vi "Pneumatic Command Initialize.vi"(11 "name (unnamed)":string) -> (2 "RTFIFO Out":u64, 3 "Cluster":T1)   [LabVIEW 2015]
uses:
  <userlib>/836-Library/Pneumatics/Support Code/Pneumatics Notifier.ctl
  <userlib>/836-Library/Pneumatics/Support Code/Pneumatics Command.ctl
  <userlib>/836-Library/Pneumatics/Support Code/Pneumatics Status.ctl
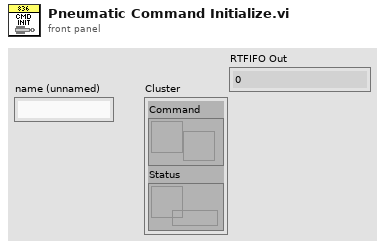
[diagram p1: front panel]
types:
  T1 = typedef "Pneumatics Notifier.ctl" = cluster{"Command":refnum<notifier>, "Status":refnum<queue>}
  T2 = typedef "Pneumatics Command.ctl" = enum16{"Nothing", "Forward", "Reverse", "Toggle"}
  T3 = typedef "Pneumatics Status.ctl" = enum16{"Forward", "Reverse", "Moving"}
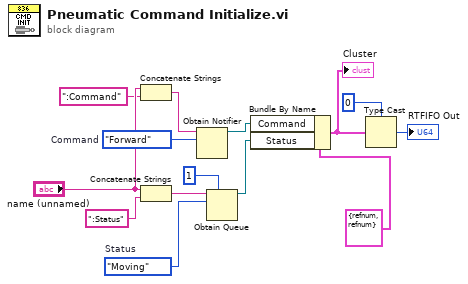
[diagram p0: block diagram]
diagram:
  w12 = Pneumatics_Command."Forward"  # Command
  w11 = Pneumatics_Status."Moving"  # Status
  n1 = Concatenate Strings("name (unnamed)", ":Command" ("string")) -> (w6:string)
  n2 = Concatenate Strings("name (unnamed)", ":Status" ("string")) -> (w9:string)
  n3 = Obtain Notifier(name (unnamed)=w6, notification data type=w12) -> (notifier out=w14:refnum<notifier>)  [unwired: 2 in, 2 out]
  n4 = Obtain Queue(max queue size (-1, unlimited)=1, name (unnamed)=w9, element data type=w11) -> (queue out=w13:refnum<queue>)  [unwired: 2 in, 2 out]
  n5 = Bundle By Name(cluster=T1 {"Command"=refnum, "Status"=refnum}, "Command"=w14, "Status"=w13) -> (w2:T1)
  "Cluster" <- w2
  n6 = Type Cast(type=u64 0, x=w2) -> (*(type *) &x=→"RTFIFO Out":u64)
